vi "Set Mutation History - NONUI.vi"(8 "error in":errorcluster, 9 "Mutation History":T1 {"LabVIEW Version" format="%.0x"}, 11 "Input object":refnum<class>) -> (0 "error out":errorcluster)   [LabVIEW 2019, in "IncrementMutationHistory.lvlib" / "VILIB_NONUI.lvlib"]
uses:
  <vilib>/Utility/EditLVLibs/LVClass/Mutation History.ctl
  <vilib>/Utility/EditLVLibs/LVClass/Mutation Record.ctl
  <vilib>/Utility/EditLVLibs/LibVersion.ctl
  VILIB_NONUI.lvlib
  <vilib>/Utility/EditLVLibs/Edit LVLibs.lvlib
panel:
  in  "error message 2":string="LabVIEW Object does not have mutation history for any class."
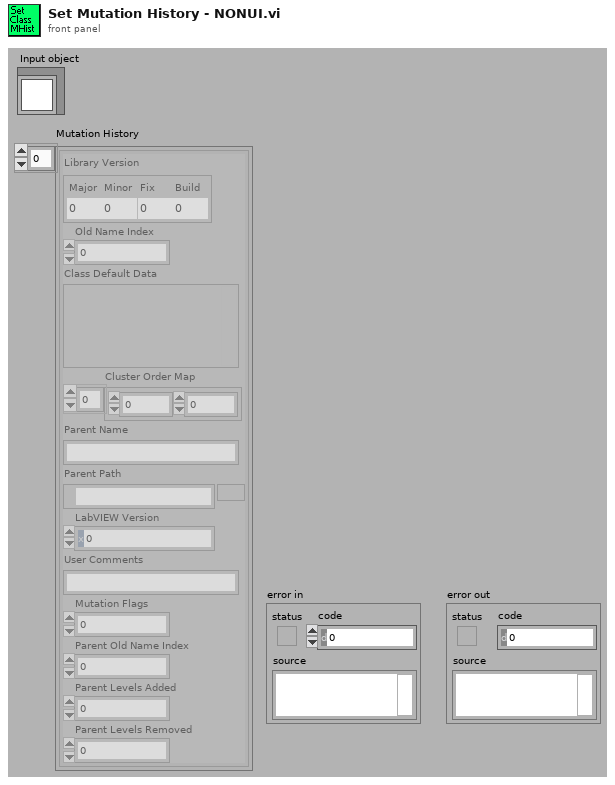
[diagram p1: front panel]
types:
  T1 = typedef "Edit LVLibs.lvlib/Mutation History.ctl" = T2[]
  T2 = typedef "Edit LVLibs.lvlib/Mutation Record.ctl" = cluster{"Library Version":T3, "Old Name Index":u8, "Class Default Data":variant, "Cluster Order Map":u32[], "Parent Name":string, "Parent Path":path, "LabVIEW Version":u32, "User Comments":string, "Mutation Flags":u8, "Parent Old Name Index":u8, "Parent Levels Added":u16, "Parent Levels Removed":u16}
  T3 = typedef "Edit LVLibs.lvlib/LibVersion.ctl" = cluster{"Major":u16, "Minor":u16, "Fix":u16, "Build":u16}
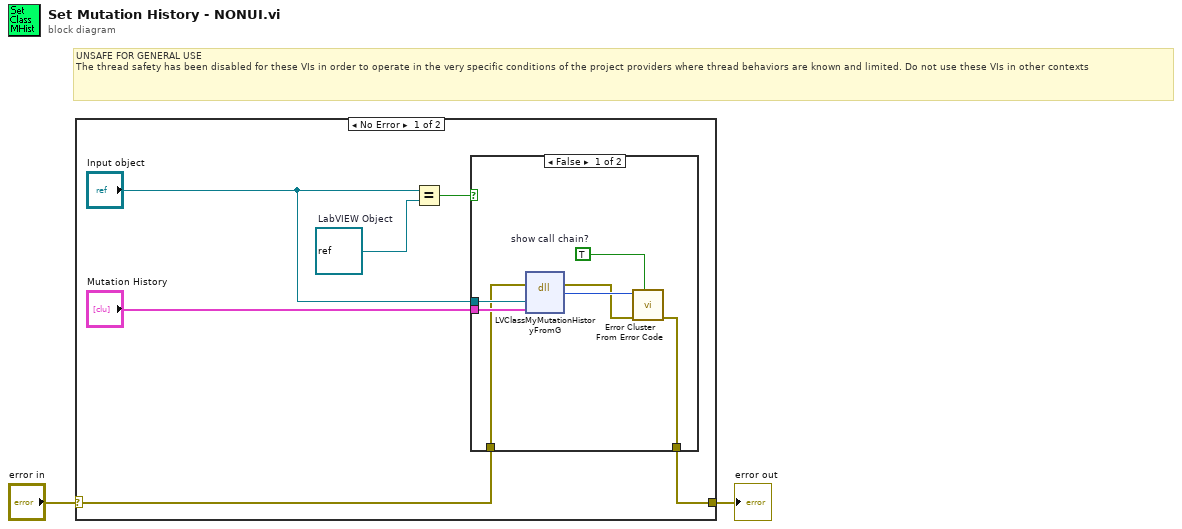
[diagram p0: block diagram]
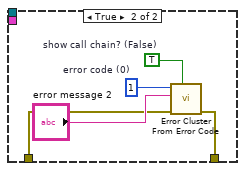
[diagram p2: hidden frame]
diagram:
  # "UNSAFE FOR GENERAL USE\nThe thread safety has been disabled for these VIs in order to operate in the very specific conditions of the project providers where thread behaviors are known and limited. Do not use these VIs in other contexts"
  n1 = case shown="No Error" "error in" {
    selector: "error in" -> [w5 w21]
    tunnel: [w6 w21] -> w1
    frame No Error {
      w4 = refnum<class> refnum  # LabVIEW Object
      n2 = Equal?(x="Input object", y=w4) -> (x = y?=w8:bool)
      n3 = case shown="False" w8 {
        tunnel: "Mutation History" -> [w12 _]
        tunnel: "Input object" -> [w13 _]
        tunnel: [w14 w17] -> w6
        tunnel: w5 -> [w9 w16]
        frame False {
          w15 = TRUE  # show call chain?
          n4 = dll-call lib="LabVIEW" fn="LVClassMyMutationHistoryFromG"(error in=w9, "object"=w13, "mutations"=w12) -> (error out=w10:errorcluster, "return type"=w11:i32)  [unwired: 4 in, 1 out]
          n5 = call <vilib>:"Error Cluster From Error Code.vi"("show call chain? (False)"=w15, "error in (no error)"=w10, "error code (0)"=w11) -> ("error out"=w14:errorcluster)  [unwired: 6 in]
        }
        frame True {
          w19 = 1  # error code (0)
          w20 = TRUE  # show call chain? (False)
          n6 = call <vilib>:"Error Cluster From Error Code.vi"("show call chain? (False)"=w20, "error in (no error)"=w16, "error message (\"\")"="error message 2", "error code (0)"=w19) -> ("error out"=w17:errorcluster)  [unwired: 5 in]
        }
      }
    }
    frame Error {
    }
  }
  "error out" <- w1
